vi "Time_loop.vi"() -> ()   [LabVIEW 2019]
uses:
  <vilib>/Platform/TimedLoop/XDataNode/timing_clust.ctl
  <vilib>/Platform/TimedLoop/XDataNode/nitl_modes.ctl
  <vilib>/Platform/TimedLoop/XDataNode/wakeup.ctl
  <vilib>/Platform/TimedLoop/scheduler/LVUserAPI/_suppVIs/Create_1kHz_TSource.vi
  <vilib>/Platform/TimedLoop/XDataNode/XDataNode.xnode
  <vilib>/Platform/TimedLoop/XDataNode/XDNodeRunTimeDep.lvlib
panel:
  out "STOP-variable":bool
  out "Nr petli głównej":i32
  out "TG - różnica czasów GLOBAL [ms]":dbl format="%.3f"
  out "TE - różnica czasów END [ms]":dbl
  in  "T1 - czas trwania pierwszej pętli [s]":dbl caption="Delay Time (s)" min=0.0 step=0.05
  in  "Czas\nspodziewany        aktualny":bool=TRUE
  out "TS - różnica czasów START [ms]":dbl
  in  "D1 - opóźnienie drugiej pętli [s]":sgl step=0.5
  in  "N - liczba iteracji":u16=1 min=1
  in  "T - okres pętli czasowych [ms]":u32
  in  "STOP":bool
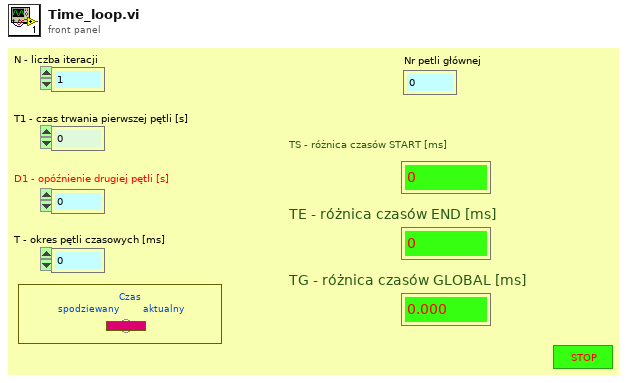
[diagram p1: front panel]
types:
  T1 = typedef "XDNodeRunTimeDep.lvlib/timing_clust.ctl" = cluster{"Expected End [f-1]":u64, "Actual End [f-1]":u64, "Finished Late? [f-1]":bool, "Expected End [i-1]":u64, "Actual End [i-1]":u64, "Finished Late? [i-1]":bool, "Expected Start [i]":u64, "Actual Start [i]":u64, "Expected Start [f]":u64, "Actual Start [f]":u64, "Source Name":string, "Structure Name":string, "Period":i64, "Deadline":i64, "Offset":i64, "Start":i64, "Priority":i32, "Timeout":i32, "Mode":T2, "Wakeup Reason":T3, "Error":errorcluster, "Source Type":string, "Secondary Source Type":string, "Global End Time":u64, "Global Start Time":u64, "Frame Duration":u64, "Iteration Duration":u64, "Assigned CPU":i32, "I/O Scan Engine Mode":u32}
  T2 = typedef "XDNodeRunTimeDep.lvlib/nitl_modes.ctl" = enum32{"No Change", "Process missed periods, maintain original phase", "Discard missed periods, maintain original phase", "Process missed periods, ignore original phase", "Discard missed periods, ignore original phase"}
  T3 = typedef "XDNodeRunTimeDep.lvlib/wakeup.ctl" = enum32{"Normal", "Aborted", "Asynchronous wakeup", "Timing source error", "Timed loop error", "Timeout"}
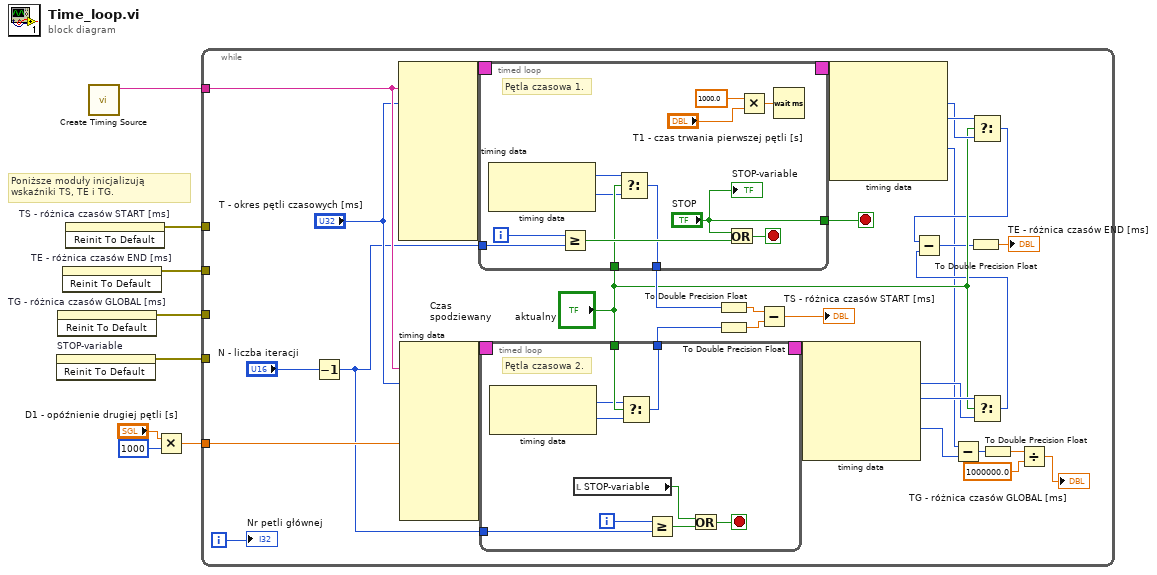
[diagram p0: block diagram]
diagram:
  # "Poniższe moduły inicjalizują \nwskaźniki TS, TE i TG."
  n1 = invoke on="STOP-variable" class="Bool (strict)" method="Reinit To Default"() -> (error out=w1:errorcluster)  [unwired: 3 in, 2 out]
  n2 = invoke on="TG - różnica czasów GLOBAL [ms]" class="DigNum (strict)" method="Reinit To Default"() -> (error out=w2:errorcluster)  [unwired: 3 in, 2 out]
  n3 = invoke on="TE - różnica czasów END [ms]" class="DigNum (strict)" method="Reinit To Default"() -> (error out=w3:errorcluster)  [unwired: 3 in, 2 out]
  n4 = invoke on="TS - różnica czasów START [ms]" class="DigNum (strict)" method="Reinit To Default"() -> (error out=w4:errorcluster)  [unwired: 3 in, 2 out]
  n5 = call-poly <vilib>:"Create Timing Source.vi"() -> ("name (out)"=w8:string)  [unwired: 10 in, 1 out]
  n6 = Multiply(x="D1 - opóźnienie drugiej pętli [s]", y=i64 1000 ("x")) -> (x*y=w5:sgl)
  n7 = while {
    tunnel: w8 -> [w35]
    tunnel: w5 -> [w34]
    tunnel: w4 -> [_]
    tunnel: w3 -> [_]
    tunnel: w2 -> [_]
    tunnel: w1 -> [_]
    i -> [w21]
    stop <- w22 stop-if-true
    n8 = Decrement(x="N - liczba iteracji") -> (x-1=w9:u16)
    n9 = node-c288(w35, "T - okres pętli czasowych [ms]") -> (w39:T1)  [unwired: 8 in]
    n10 = node-c288(w35, "T - okres pętli czasowych [ms]", w34) -> (w37:T1)  [unwired: 7 in]
    n11 = timed-loop {
      timing: w39 -> [_]
      timing-out: [_] -> w38
      tunnel: w9 -> [w73]
      tunnel: ["STOP"] -> w22
      tunnel: "Czas\nspodziewany        aktualny" -> [w70]
      tunnel: [w69] -> w33
      i -> [w68]
      stop <- w71 stop-if-true
      # "Pętla czasowa 1."
      n12 = node-c288() -> (w67:i64, w66:i64)  [unwired: 1 in]
      n13 = Greater Or Equal?(x=w68, y=w73) -> (x >= y?=w72:bool)
      n14 = Select(t=w67, s=w70, f=w66) -> (s? t:f=w69:i64)
      n15 = Or(x="STOP", y=w72) -> (x .or. y?=w71:bool)
      n16 = Multiply(x=1000.0, y="T1 - czas trwania pierwszej pętli [s]") -> (x*y=w65:dbl)
      n17 = Wait (ms)(milliseconds to wait=w65) -> ()  [unwired: 1 out]
      "STOP-variable" <- "STOP"
    }
    n18 = timed-loop {
      timing: w37 -> [_]
      timing-out: [_] -> w36
      tunnel: w9 -> [w48]
      tunnel: "Czas\nspodziewany        aktualny" -> [w46]
      tunnel: [w45] -> w32
      i -> [w47]
      stop <- w40 stop-if-true
      # "Pętla czasowa 2."
      n19 = node-c288() -> (w44:i64, w43:i64)  [unwired: 1 in]
      n20 = local read "STOP-variable"() -> (w41:bool)
      n21 = Select(t=w44, s=w46, f=w43) -> (s? t:f=w45:i64)
      n22 = Greater Or Equal?(x=w47, y=w48) -> (x >= y?=w42:bool)
      n23 = Or(x=w41, y=w42) -> (x .or. y?=w40:bool)
    }
    n24 = To Double Precision Float(number=w33) -> (double precision float=w16:dbl)
    n25 = To Double Precision Float(number=w32) -> (double precision float=w15:dbl)
    n26 = Subtract(x=w16, y=w15) -> (x-y=→"TS - różnica czasów START [ms]":dbl)
    n27 = node-c288(w36) -> (w30:i64, w31:i64, w11:i64)  [unwired: 3 out]
    n28 = node-c288(w38) -> (w28:i64, w29:i64, w12:i64)  [unwired: 3 out]
    n29 = Subtract(x=w12, y=w11) -> (x-y=w18:i64)
    n30 = Select(t=w29, s="Czas\nspodziewany        aktualny", f=w28) -> (s? t:f=w13:i64)
    n31 = Select(t=w31, s="Czas\nspodziewany        aktualny", f=w30) -> (s? t:f=w14:i64)
    n32 = Subtract(x=w13, y=w14) -> (x-y=w20:i64)
    n33 = To Double Precision Float(number=w20) -> (double precision float=→"TE - różnica czasów END [ms]":dbl)
    n34 = To Double Precision Float(number=w18) -> (double precision float=w17:dbl)
    n35 = Divide(x=w17, y=1000000.0) -> (x/y=→"TG - różnica czasów GLOBAL [ms]":dbl)
    "Nr petli głównej" <- w21
  }
